vi "运维调试_其他.vi"() -> ()   [LabVIEW 2016, in "其他.lvlib"]
uses:
  <vilib>/Utility/miscctls.llb/LVPointTypeDef.ctl
  PLC/PLC.lvlib
  <vilib>/ptbypt/NI_PtbyPt.lvlib
panel:
  out "集成报警信息":string
  out "R115":i16 caption="灯带关闭时间"
  out "R114":i16 caption="灯带开启时间"
  in  "视频监控":bool
  in  "照明":bool
  in  "前门灯带":bool
  in  "侧边灯带":bool
  # "H"
  # "H"
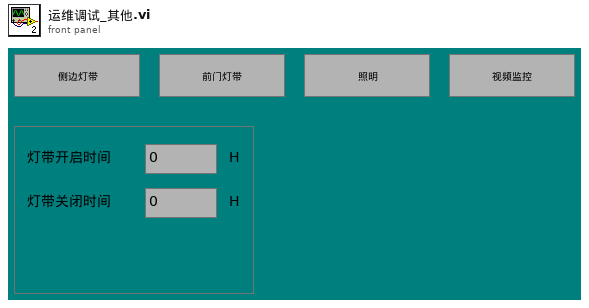
[diagram p1: front panel]
types:
  T1 = cluster{"R100":i16, "R101":i16, "R102":i16, "R103":i16, "R104":i16, "R105":i16, "R106":i16, "R107":i16, "R108":i16, "R109":i16, "R110":i16, "R111":i16, "R112":i16, "R113":i16, "R114":i16, "R115":i16, "R116":i16, "R117":i16, "R118":i16, "R119":i16}
  T2 = typedef "LVPointTypeDef.ctl" = cluster{"Horizontal":i16, "Vertical":i16}
  T3 = cluster{"命令":string, "data":cluster{"starting address":u16, "coil values":bool[]}}
  T4 = cluster{"命令":string, "数据":cluster{"starting address":u16, "holding register values":u16[]}}
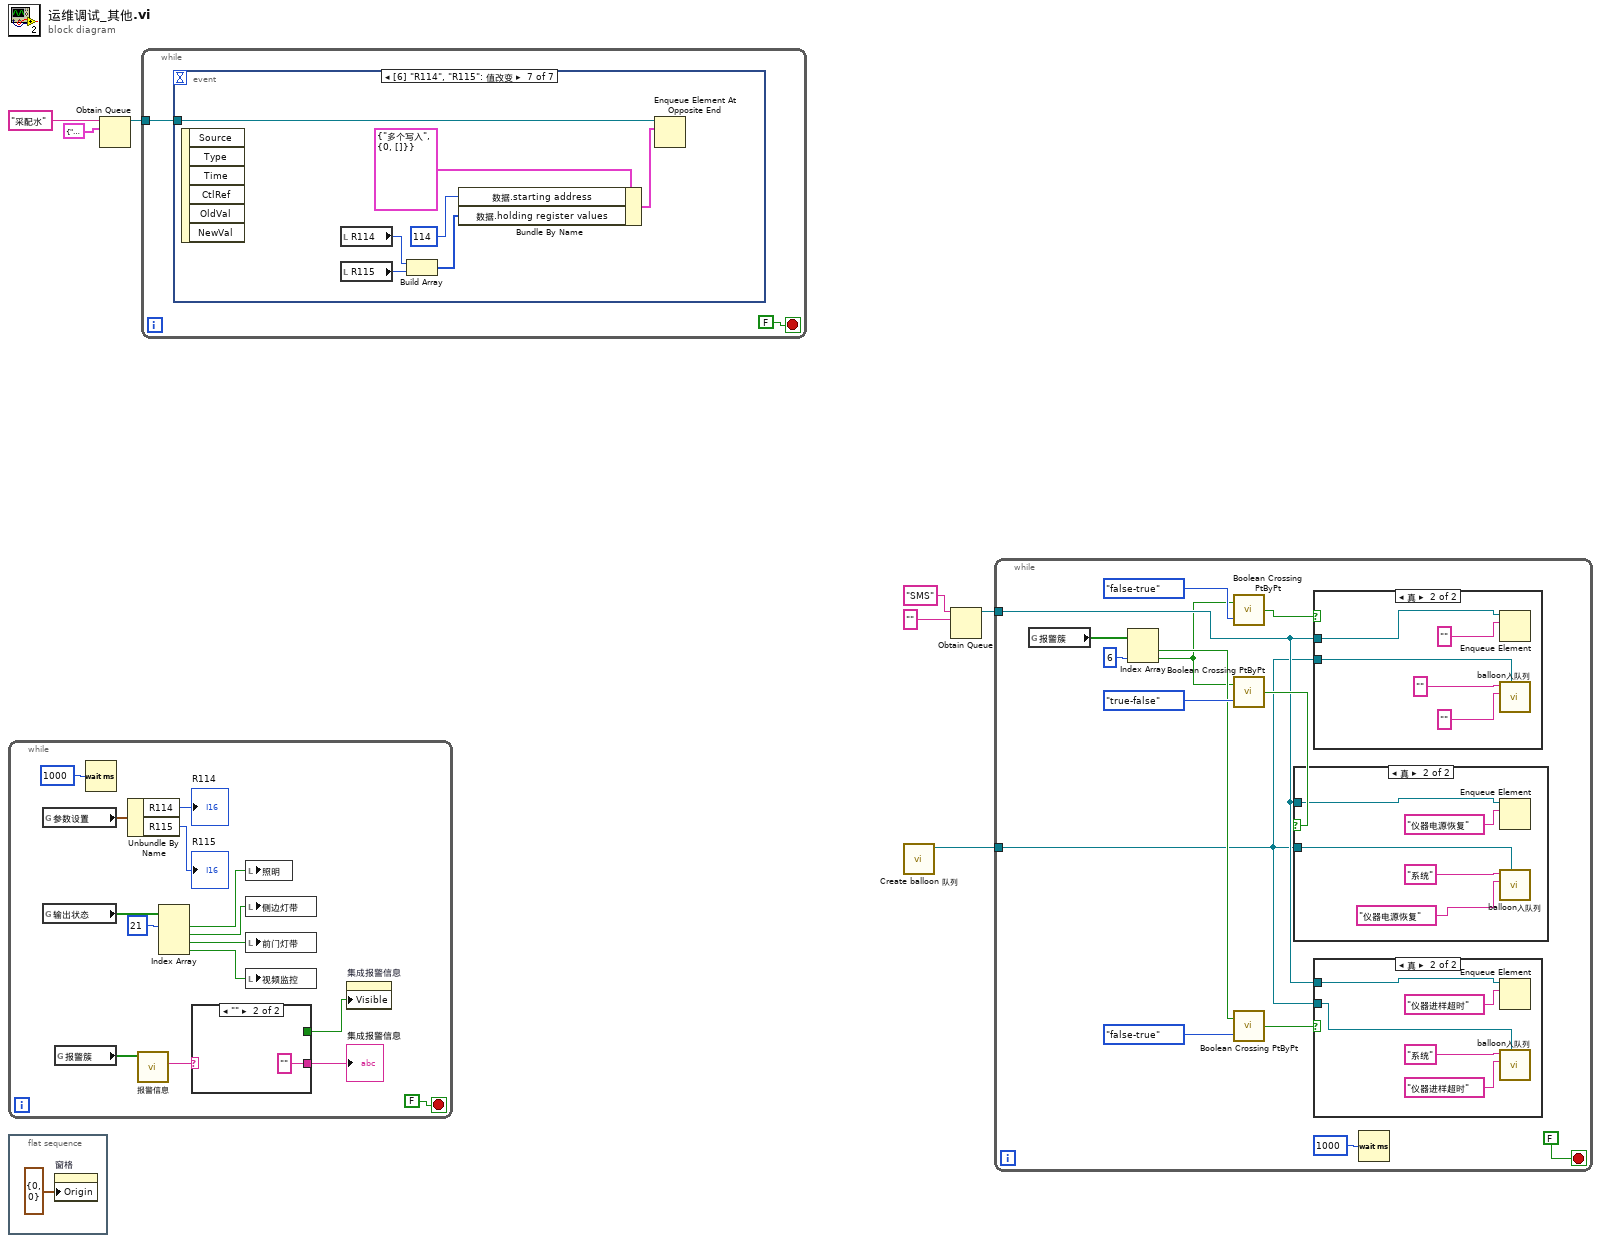
[diagram p0: block diagram]
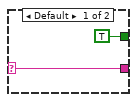
[diagram p5: hidden frame]
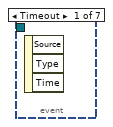
[diagram p6: hidden frame]
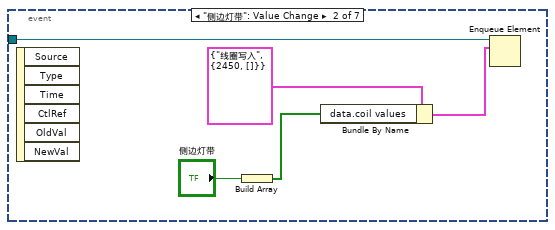
[diagram p7: hidden frame]
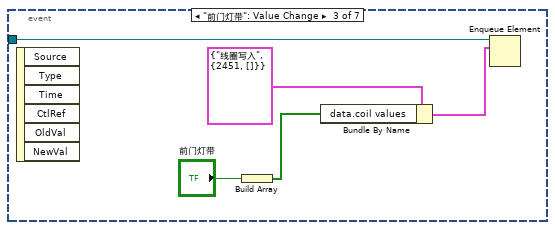
[diagram p8: hidden frame]
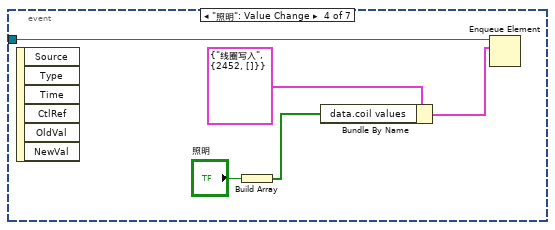
[diagram p9: hidden frame]
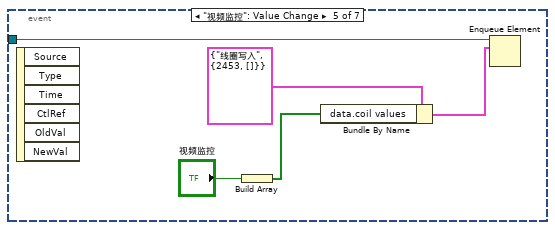
[diagram p10: hidden frame]
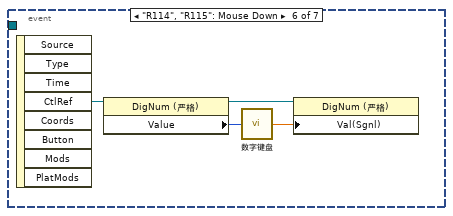
[diagram p11: hidden frame]
diagram:
  n1 = while {
    stop <- FALSE stop-if-true
    n2 = global read "采配水全局变量.vi" "参数设置"() -> (w20:T1)
    n3 = global read "采配水全局变量.vi" "输出状态"() -> (w13:bool[])
    n4 = global read "采配水全局变量.vi" "报警簇"() -> (w14:bool[])
    n5 = Wait (ms)(milliseconds to wait=u32 1000 ("等待时间（毫秒）")) -> ()  [unwired: 1 out]
    n6 = Unbundle By Name(w20) -> ("R114"=→"R114":i16, "R115"=→"R115":i16)
    n7 = call "报警信息.vi"("报警簇"=w14) -> ("系统报警信息"=w17:string)  [unwired: 9 in, 1 out]
    n8 = Index Array(array=w13, index #1=21 ("索引")) -> (element #1=w11:bool, element #2=w10:bool, element #3=w12:bool, element #4=w9:bool)  [unwired: 3 in]
    n9 = case shown="\"\"" w17 {
      selector: w17 -> [w24 _]
      tunnel: [w24 "" ("字符串")] -> w15
      tunnel: [TRUE ("可见") _] -> w16
      frame Default {
      }
      frame "" {
      }
    }
    "集成报警信息" <- w15
    n10 = local write "照明"(w11) -> ()
    n11 = local write "侧边灯带"(w10) -> ()
    n12 = local write "前门灯带"(w12) -> ()
    n13 = local write "视频监控"(w9) -> ()
    n14 = property on="集成报警信息" class="Str"("Visible"=w16) -> ()  [unwired: 2 in, 2 out]
  }
  n15 = flat-sequence {
    frame #0 {
      n16 = property on="窗格" class="Pane"("Origin"=T2 {"Horizontal"=0, "Vertical"=0} ("原点")) -> ()  [unwired: 2 in, 2 out]
    }
  }
  n17 = Obtain Queue(name (unnamed)="采配水" ("名称（未命名）"), element data type=cluster{"命令":string, "数据":variant} {"命令"="", "数据"=variant}) -> (queue out=w5:refnum<queue>)  [unwired: 3 in, 2 out]
  n18 = while {
    tunnel: w5 -> [w27]
    stop <- FALSE stop-if-true
    n19 = event shown="[6] \"R114\", \"R115\": 值改变" {
      selector: _ -> [_ _ _ _ _ _ _]
      dyn-events: _ -> [_ _ _ _ _ _ _]
      timeout: _ -> [_ _ _ _ _ _ _]
      tunnel: w27 -> [_ w30 w36 w41 w46 _ w53]
      event Timeout {
        n20 = event-data() -> ()  [unwired: 1 in, 3 out]
      }
      event "侧边灯带": Value Change {
        n21 = event-data() -> ()  [unwired: 1 in, 6 out]
        n22 = Build Array("侧边灯带") -> (w29:bool[])
        n23 = Bundle By Name(cluster=T3 {"命令"="线圈写入", "data"={"starting address"=2450, "coil values"=[]}} ("元素"), "data.coil values"=w29) -> (w31:T3)
        n24 = Enqueue Element(queue=w30, element=w31) -> ()  [unwired: 2 in, 3 out]
      }
      event "前门灯带": Value Change {
        n25 = event-data() -> ()  [unwired: 1 in, 6 out]
        n26 = Build Array("前门灯带") -> (w35:bool[])
        n27 = Bundle By Name(cluster=T3 {"命令"="线圈写入", "data"={"starting address"=2451, "coil values"=[]}} ("元素"), "data.coil values"=w35) -> (w37:T3)
        n28 = Enqueue Element(queue=w36, element=w37) -> ()  [unwired: 2 in, 3 out]
      }
      event "照明": Value Change {
        n29 = event-data() -> ()  [unwired: 1 in, 6 out]
        n30 = Build Array("照明") -> (w40:bool[])
        n31 = Bundle By Name(cluster=T3 {"命令"="线圈写入", "data"={"starting address"=2452, "coil values"=[]}} ("元素"), "data.coil values"=w40) -> (w42:T3)
        n32 = Enqueue Element(queue=w41, element=w42) -> ()  [unwired: 2 in, 3 out]
      }
      event "视频监控": Value Change {
        n33 = event-data() -> ()  [unwired: 1 in, 6 out]
        n34 = Build Array("视频监控") -> (w45:bool[])
        n35 = Bundle By Name(cluster=T3 {"命令"="线圈写入", "data"={"starting address"=2453, "coil values"=[]}} ("元素"), "data.coil values"=w45) -> (w47:T3)
        n36 = Enqueue Element(queue=w46, element=w47) -> ()  [unwired: 2 in, 3 out]
      }
      event "R114", "R115": Mouse Down {
        n37 = event-data() -> ("CtlRef"=w52:refnum<vi>)  [unwired: 1 in, 7 out]
        n38 = property class="DigNum (严格)"(reference=w52) -> (reference out=w51:refnum<vi>, "Value"=w50:i16)  [unwired: 1 in, 1 out]
        n39 = call "数字键盘.vi"("OldNumber"=w50) -> ("NewNumber"=w49:sgl)
        n40 = property class="DigNum (严格)"(reference=w51, "Val(Sgnl)"=w49) -> ()  [unwired: 1 in, 2 out]
      }
      event "R114", "R115": Value Change {
        n41 = event-data() -> ()  [unwired: 1 in, 6 out]
        n42 = local read "R114"() -> (w58:i16)
        n43 = local read "R115"() -> (w59:i16)
        n44 = Build Array(w58, w59) -> (w54:i16[])
        n45 = Bundle By Name(cluster=T4 {"命令"="多个写入", "数据"={"starting address"=0, "holding register values"=[]}} ("元素"), "数据.starting address"=u16 114, "数据.holding register values"=w54) -> (w55:T4)
        n46 = Enqueue Element At Opposite End(queue=w53, element=w55) -> ()  [unwired: 2 in, 3 out]
      }
    }
  }
  n47 = call "Create balloon 队列.vi"() -> ("队列输出"=w1:refnum<queue>)  [unwired: 11 in]
  n48 = Obtain Queue(name (unnamed)="SMS" ("名称（未命名）"), element data type="" ("名称（未命名）")) -> (queue out=w2:refnum<queue>)  [unwired: 3 in, 2 out]
  n49 = while {
    tunnel: w2 -> [w67]
    tunnel: w1 -> [w60]
    stop <- FALSE stop-if-true
    n50 = global read "采配水全局变量.vi" "报警簇"() -> (w64:bool[])
    n51 = Index Array(array=w64, index #2=6 ("索引")) -> (element #1=w63:bool, element #2=w61:bool)  [unwired: 1 in]
    n52 = call <vilib>:"Boolean Crossing PtByPt.vi"("direction"=enum16{"either", "false-true", "true-false"}."false-true", "input"=w61) -> ("crossing"=w70:bool)  [unwired: 1 in]
    n53 = call <vilib>:"Boolean Crossing PtByPt.vi"("direction"=enum16{"either", "false-true", "true-false"}."true-false", "input"=w61) -> ("crossing"=w68:bool)  [unwired: 1 in]
    n54 = call <vilib>:"Boolean Crossing PtByPt.vi"("direction"=enum16{"either", "false-true", "true-false"}."false-true", "input"=w63) -> ("crossing"=w65:bool)  [unwired: 1 in]
    n55 = case shown="真" w68 {
      tunnel: w67 -> [_ w81]
      tunnel: w60 -> [_ w80]
      frame False {
      }
      frame True {
        n56 = Enqueue Element(queue=w81, element="仪器电源恢复" ("元素")) -> ()  [unwired: 2 in, 3 out]
        n57 = call "balloon入队列.vi"("队列"=w80, "故障信息"="仪器电源恢复" ("元素"), "参数名称"="系统") -> ()  [unwired: 8 in, 1 out]
      }
    }
    n58 = case shown="真" w70 {
      tunnel: w67 -> [_ w88]
      tunnel: w60 -> [_ w86]
      frame False {
      }
      frame True {
        n59 = Enqueue Element(queue=w88, element="" ("元素")) -> ()  [unwired: 2 in, 3 out]
        n60 = call "balloon入队列.vi"("队列"=w86, "故障信息"="" ("元素"), "参数名称"="") -> ()  [unwired: 8 in, 1 out]
      }
    }
    n61 = case shown="真" w65 {
      tunnel: w67 -> [_ w78]
      tunnel: w60 -> [_ w76]
      frame False {
      }
      frame True {
        n62 = Enqueue Element(queue=w78, element="仪器进样超时" ("元素")) -> ()  [unwired: 2 in, 3 out]
        n63 = call "balloon入队列.vi"("队列"=w76, "故障信息"="仪器进样超时" ("元素"), "参数名称"="系统") -> ()  [unwired: 8 in, 1 out]
      }
    }
    n64 = Wait (ms)(milliseconds to wait=u32 1000 ("等待时间（毫秒）")) -> ()  [unwired: 1 out]
  }
